vi "Write AO Data.vi"(8 "error in (no error)":errorcluster, 10 "AO Data":dbl[](array[numeric]), 11 "BNT_DAQmx-MCSV-Data in":refnum<class "BNT_DAQmx-MCSV-Data.lvclass">) -> (0 "error out":errorcluster, 3 "BNT_DAQmx-MCSV-Data out":refnum<class "BNT_DAQmx-MCSV-Data.lvclass">)   [LabVIEW 2021, in "BNT_DAQmx.lvlib" / "BNT_DAQmx-MCSV-Data.lvclass"]
doc: "Write AO data."
uses:
  BNT_DAQmx-MCSV-Data.lvclass
  BNT_DAQmx-MCSV-Data.lvclass/BNT_DAQmx-MCSV-Data.ctl
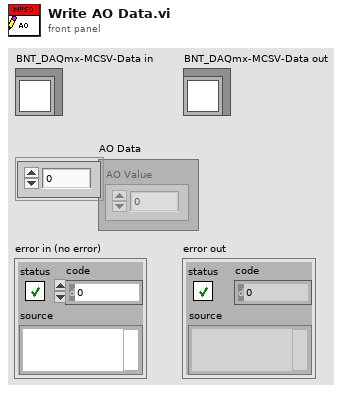
[diagram p1: front panel]
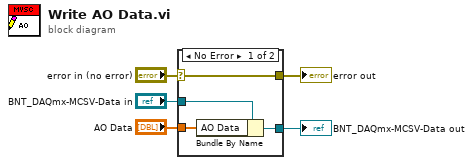
[diagram p0: block diagram]
diagram:
  n1 = case shown="No Error" "error in (no error)" {
    selector: "error in (no error)" -> [w9 w10]
    tunnel: [w9 w10] -> w4
    tunnel: [w7 w11] -> w2
    tunnel: "BNT_DAQmx-MCSV-Data in" -> [w8 w11]
    tunnel: "AO Data" -> [w6 _]
    frame No Error {
      n2 = Bundle By Name(cluster=w8, "AO Data"=w6) -> (w7:refnum<class "BNT_DAQmx-MCSV-Data.lvclass">)
    }
    frame Error {
    }
  }
  "error out" <- w4
  "BNT_DAQmx-MCSV-Data out" <- w2
